vi "去空格.vi"(10 "Array":string[](array[string]), 11 "String":string) -> (2 "Array out":string[](array[string]), 3 "result string":string)   [LabVIEW 2016]
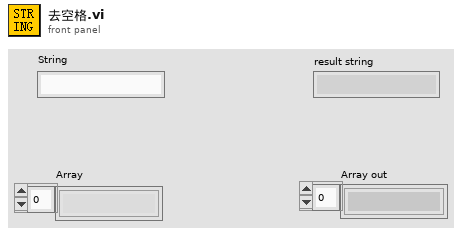
[diagram p1: front panel]
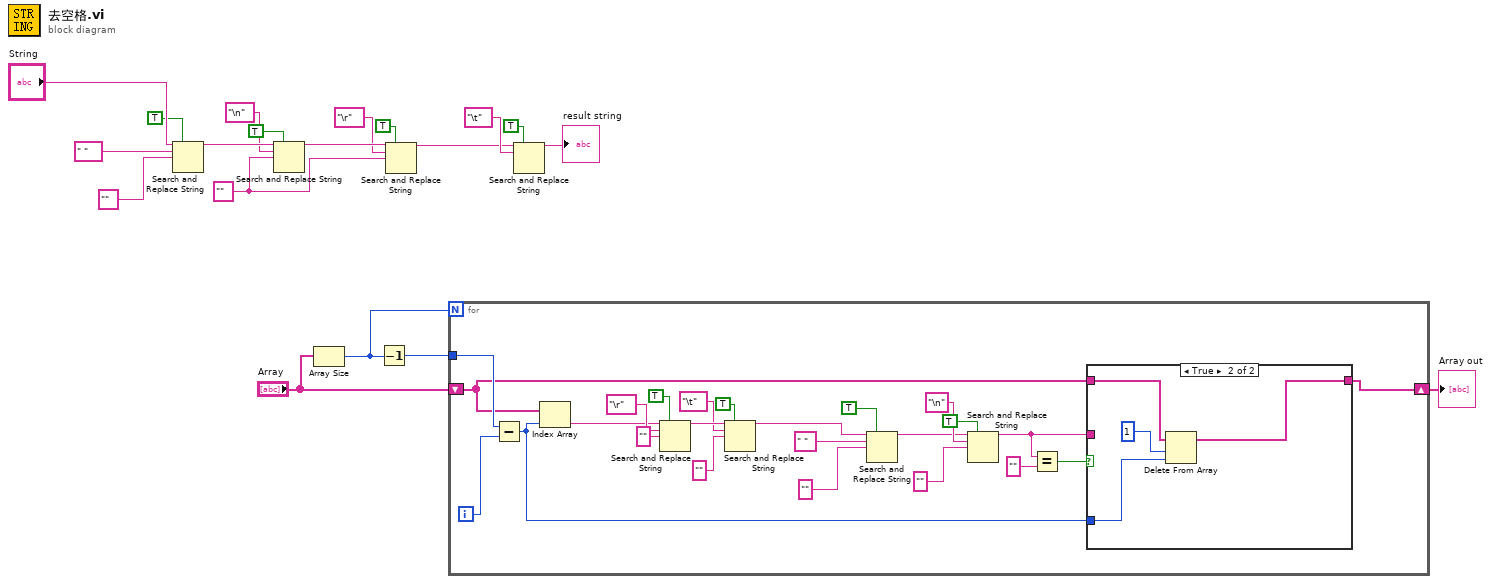
[diagram p0: block diagram]
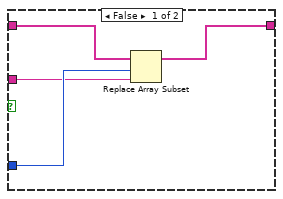
[diagram p2: hidden frame]
diagram:
  w7 = "" ("replace string (\"\")")
  n1 = Search and Replace String(replace all?=TRUE ("replace all? (F)"), input string="String", search string=" ", replace string="" ("replace string (\"\")")) -> (result string=w16:string)  [unwired: 4 in, 3 out]
  n2 = Search and Replace String(replace all?=TRUE ("replace all? (F)"), input string=w16, search string="\n", replace string=w7) -> (result string=w8:string)  [unwired: 4 in, 3 out]
  n3 = Array Size(array="Array") -> (size(s)=w11:i32)
  n4 = Decrement(x=w11) -> (x-1=w10:i32)
  n5 = Search and Replace String(replace all?=TRUE ("replace all? (F)"), input string=w8, search string="\r", replace string=w7) -> (result string=w2:string)  [unwired: 4 in, 3 out]
  n6 = for {
    N: w11 -> [_]
    shift-right: [w30] -> w9
    shift-left: "Array" -> [w32]
    tunnel: w10 -> [w43]
    i -> [w42]
    n7 = Subtract(x=w43, y=w42) -> (x-y=w31:i32)
    n8 = Index Array(array=w32, index=w31) -> (element=w26:string)
    n9 = Search and Replace String(replace all?=TRUE ("replace all? (F)"), input string=w26, search string="\r", replace string="" ("replace string (\"\")")) -> (result string=w24:string)  [unwired: 4 in, 3 out]
    n10 = Search and Replace String(replace all?=TRUE ("replace all? (F)"), input string=w24, search string="\t", replace string="" ("replace string (\"\")")) -> (result string=w22:string)  [unwired: 4 in, 3 out]
    n11 = Search and Replace String(replace all?=TRUE ("replace all? (F)"), input string=w22, search string=" ", replace string="" ("replace string (\"\")")) -> (result string=w37:string)  [unwired: 4 in, 3 out]
    n12 = Search and Replace String(replace all?=TRUE ("replace all? (F)"), input string=w37, search string="\n", replace string="" ("replace string (\"\")")) -> (result string=w29:string)  [unwired: 4 in, 3 out]
    n13 = Equal?(x=w29, y="") -> (x = y?=w33:bool)
    n14 = case shown="True" w33 {
      tunnel: w32 -> [w47 w51]
      tunnel: w31 -> [w46 w50]
      tunnel: [w44 w48] -> w30
      tunnel: w29 -> [w45 _]
      frame False {
        n15 = Replace Array Subset(array=w47, new element=w45, index=w46) -> (w44:string[])
      }
      frame True {
        n16 = Delete From Array(array=w51, length=1, index=w50) -> (array with subset deleted=w48:string[])  [unwired: 1 out]
      }
    }
  }
  "Array out" <- w9
  n17 = Search and Replace String(replace all?=TRUE ("replace all? (F)"), input string=w2, search string="\t") -> (result string=→"result string":string)  [unwired: 5 in, 3 out]
